vi "NI VeriStand - Add Child Nodes.vi"(8 "Error in":errorcluster, 10 "Child Nodes":u64[](array[numeric]), 11 "Runtime Configuration Ref in":refnum<k39>) -> (0 "Error out":errorcluster, 2 "Success":bool, 3 "Runtime Configuration Ref out":refnum<k39>)   [LabVIEW 2027, in "Runtime Configuration File API.lvlib"]
uses:
  Runtime Configuration File API.lvlib
  C:/NetCoreDLL/NationalInstruments.VeriStand.SystemDefinitionAPI.dll
  NetCoreDLL/NationalInstruments.VeriStand.SystemDefinitionAPI.dll
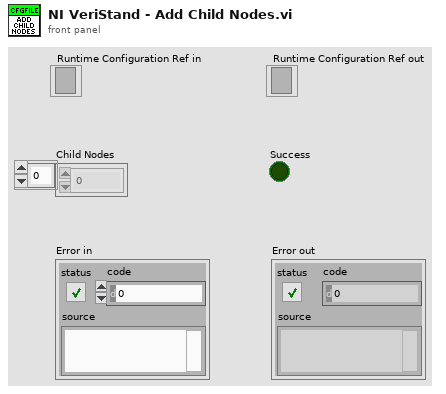
[diagram p1: front panel]
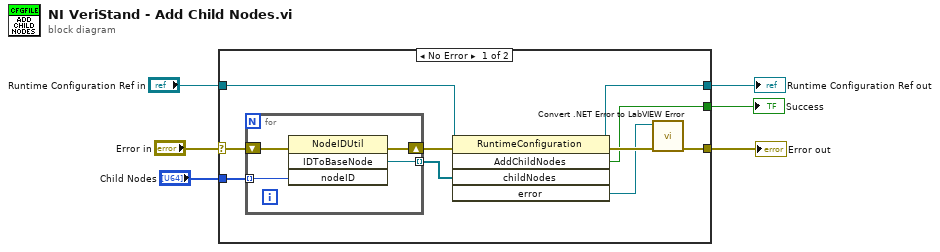
[diagram p0: block diagram]
diagram:
  n1 = case shown="No Error" "Error in" {
    selector: "Error in" -> [w16 _]
    tunnel: "Runtime Configuration Ref in" -> [w12 w21]
    tunnel: [w11 w21] -> w3
    tunnel: [w13 _] -> w6
    tunnel: "Child Nodes" -> [w10 _]
    tunnel: [w8 _] -> w1
    frame No Error {
      n2 = for {
        tunnel: w10 -> [w18] mode=indexing
        shift-right: [w19] -> w15
        shift-left: w16 -> [w20]
        tunnel: [w17] -> w9 mode=indexing
        n3 = invoke class="NodeIDUtil" method="IDToBaseNode"(error in=w20, "nodeID"=w18) -> (error out=w19:errorcluster, "IDToBaseNode"=w17:refnum<k39>)  [unwired: 2 in, 2 out]
      }
      n4 = invoke class="RuntimeConfiguration" method="AddChildNodes"(reference=w12, error in=w15, "childNodes"=w9) -> (reference out=w11:refnum<k39>, error out=w14:errorcluster, "AddChildNodes"=w8:bool, "error"=w7:refnum<k39>)  [unwired: 2 in, 1 out]
      n5 = call "Convert .NET Error to LabVIEW Error.vi"("error in"=w14, "NationalInstruments.VeriStand.Error"=w7) -> ("error out"=w13:errorcluster)  [unwired: 9 in]
    }
    frame Error {
    }
  }
  "Runtime Configuration Ref out" <- w3
  "Success" <- w1
  "Error out" <- w6
